vi "BroadcastModuleStopStatusUpdate.vi"(8 "error in":errorcluster, 11 "Module Name in":string) -> (0 "error out":errorcluster, 3 "Module Name out":string)   [LabVIEW 2018]
uses:
  NistPluggableModules/Visualization/VisualizeBase/VisualizeBase_class/VisualizeBase.lvclass
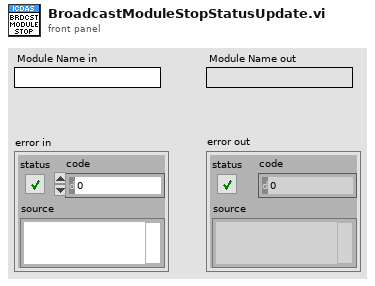
[diagram p1: front panel]
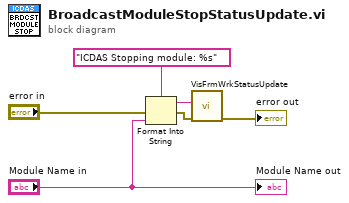
[diagram p0: block diagram]
diagram:
  n1 = Format Into String(format string="ICDAS Stopping module: %s", error in="error in", "Module Name in") -> (resulting string=w4:string, error out=w2:errorcluster)  [unwired: 1 in]
  n2 = call "VisFrmWrkStatusUpdate.vi"("error in (no error)"=w2, "Status"=w4) -> ("error out"=→"error out":errorcluster)  [unwired: 9 in]
  "Module Name out" <- "Module Name in"
